vi "LEDs immediate.vi"(7 "Description":string, 8 "Command Info In":T2, 9 "Operation":T1, 10 "seizure active":bool, 11 "Setpoint":dbl) -> (0 "Command Info Out":T2)   [LabVIEW 2019]
doc: "This template is useful for immediate subsystem actions that do not need deadband filtering\n\nBe sure to right-click and select New from Template and save with a new command name."
uses:
  <vilib>/Rock Robotics/WPI/Framework/Command Status Info.ctl
  <vilib>/Rock Robotics/WPI/Framework/Completion Status.ctl
  <vilib>/Rock Robotics/WPI/Framework/Completion Notifier.ctl
  Implementation/LEDS Operations.ctl
  Implementation/LEDS Setpoints.ctl
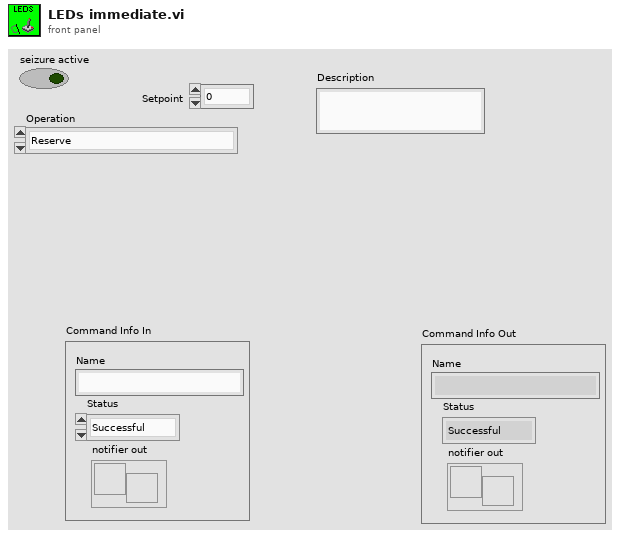
[diagram p1: front panel]
types:
  T1 = typedef "LEDS Operations.ctl" = enum16{"Reserve", "Read Current", "Immediate", "Seizure-inducing"}
  T2 = typedef "Command Status Info.ctl" = cluster{"Name":string, "Status":T3, "notifier out":T4}
  T3 = typedef "Completion Status.ctl" = enum16{"Successful", "Aborted", "Incomplete"}
  T4 = typedef "Completion Notifier.ctl" = refnum<notifier>
  T5 = typedef "LEDS Setpoints.ctl" = cluster{"Operation":T1, "Setpoint":dbl, "Duration":dbl, "seizure active":bool, "pwmOutput":dbl}
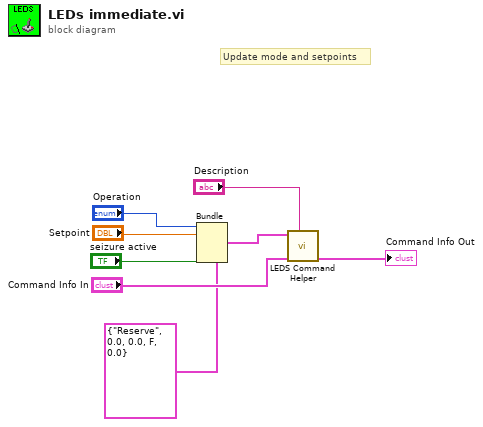
[diagram p0: block diagram]
diagram:
  # "Update mode and setpoints"
  n1 = Bundle(cluster=T5 {"Operation"=enum."Reserve", "Setpoint"=0.0, "Duration"=0.0, "seizure active"=FALSE, "pwmOutput"=0.0} ("SubSystem Data"), "Operation"="Operation", "Setpoint"="Setpoint", "seizure active"="seizure active") -> (w3:T5)  [unwired: 2 in]
  n2 = call "LEDS Command Helper.vi"("Description"="Description", "Command Info In"="Command Info In", "SubSystem Data"=w3) -> ("Command Info Out"=→"Command Info Out":T2)  [unwired: 6 in, 2 out]
